vi "CC_Get.vi"(8 "error in (no error)":errorcluster, 11 "Agilis in":T1) -> (0 "error out":errorcluster, 2 "Channel Number":i32, 3 "Agilis out":T1)   [LabVIEW 2016, in "Drivers.lvlib" / "Agilis.lvlib"]
doc: "This command is specific to AG-UC8. The piezo actuators are selected by paris which are grouped in four channels. This command <b>query</b> the selected channel."
uses:
  Agilis.lvlib
  AgilisCmdLib Refnum.ctl
  Z:/TraceGrabber/Drivers/Agilis/AgilisCmdLib.dll
  AgilisCmdLib.dll
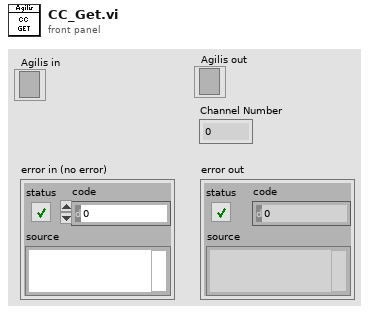
[diagram p1: front panel]
types:
  T1 = typedef "Drivers.lvlib/Agilis.lvlib/AgilisCmdLib Refnum.ctl" = refnum<k24>
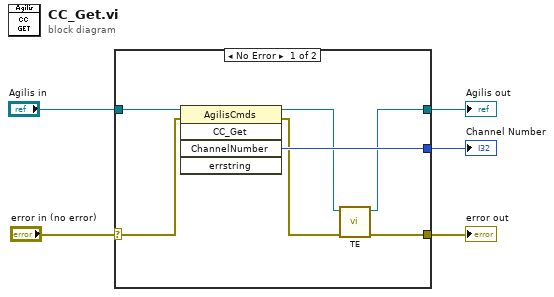
[diagram p0: block diagram]
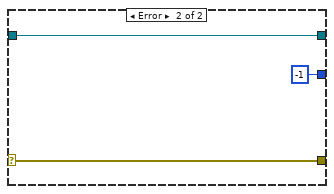
[diagram p2: hidden frame]
diagram:
  n1 = case shown="No Error" "error in (no error)" {
    selector: "error in (no error)" -> [w11 w15]
    tunnel: "Agilis in" -> [w12 w14]
    tunnel: [w8 w14] -> w3
    tunnel: [w9 w15] -> w2
    tunnel: [w10 -1 ("ChannelNumber")] -> w1
    frame No Error {
      n2 = invoke class="AgilisCmds" method="CC_Get"(reference=w12, error in=w11) -> (reference out=w7:T1, error out=w6:errorcluster, "ChannelNumber"=w10:i32)  [unwired: 3 in, 2 out]
      n3 = call "TE.vi"("error in (no error)"=w6, "Agilis in"=w7) -> ("error out"=w9:errorcluster, "Agilis out"=w8:T1)  [unwired: 8 in]
    }
    frame Error {
    }
  }
  "Agilis out" <- w3
  "error out" <- w2
  "Channel Number" <- w1
